vi "Save Animated GIF To File (Core).vi"(7 "Dither (None)":T2, 8 "error in (no error)":errorcluster, 9 "Delays":i32[](array[numeric]), 10 "Frames":T1[](array[typedef]), 11 "Path In":string) -> (0 "error out":errorcluster, 3 "Path Out":string)   [LabVIEW 2020, in "G-Image.lvlib"]
doc: "Saves an image in GIF format to disk."
uses:
  G-Image.lvlib
  Controls/Dither Type.ctl
  <vilib>/picture/picture.llb/imagedata.ctl
  Private/ARGB To RGBA.vi
  Private/Depth To Number Channels.vi
  <vilib>/Utility/error.llb/Error Cluster From Error Code.vi
  lib/g_image_32.dll
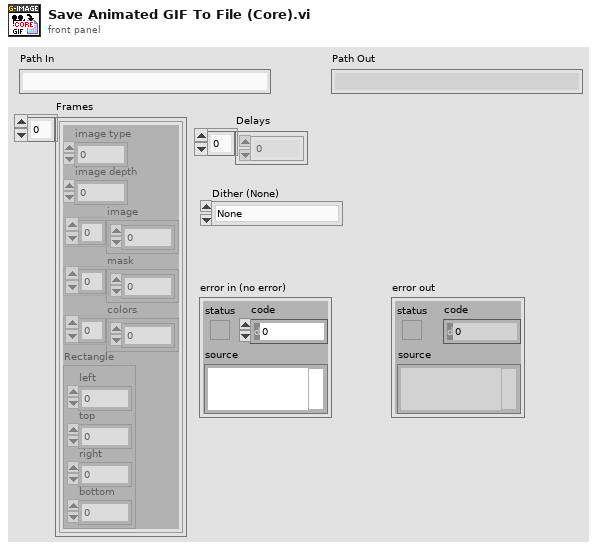
[diagram p1: front panel]
types:
  T1 = typedef "imagedata.ctl" = cluster{"image type":i32, "image depth":i32, "image":u8[], "mask":u8[], "colors":u32[], "Rectangle":cluster{"left":i16, "top":i16, "right":i16, "bottom":i16}}
  T2 = typedef "G-Image.lvlib/Dither Type.ctl" = enum32{"None", "Floyd-Steinberg"}
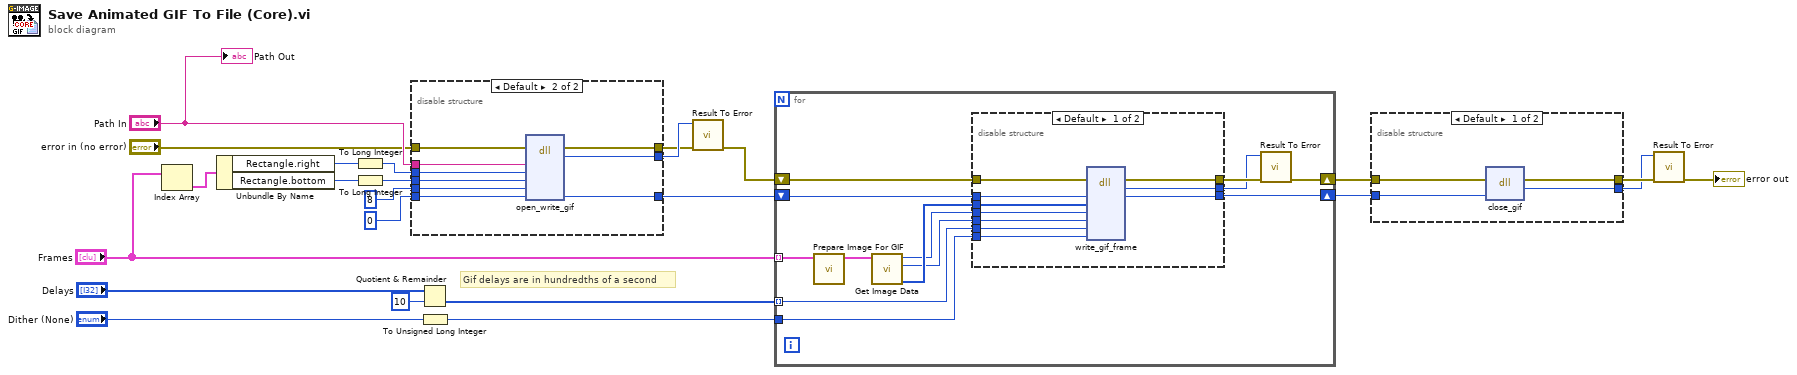
[diagram p0: block diagram]
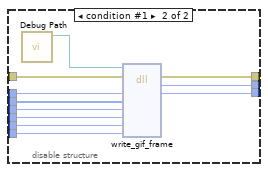
[diagram p2: hidden frame]
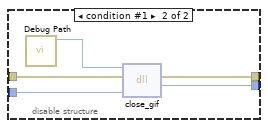
[diagram p3: hidden frame]
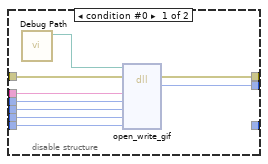
[diagram p4: hidden frame]
diagram:
  # "Gif delays are in hundredths of a second"
  n1 = Index Array(array="Frames") -> (element=w21:T1)  [unwired: 1 in]
  n2 = Unbundle By Name(w21) -> ("Rectangle.right"=w20:i16, "Rectangle.bottom"=w18:i16)
  n3 = To Long Integer(number=w20) -> (32bit integer=w19:i32)
  n4 = To Long Integer(number=w18) -> (32bit integer=w17:i32)
  n5 = disable-structure shown="Default" {
    disable-tunnel: [w33 w42] -> w22
    disable-tunnel: "error in (no error)" -> [w32 w41]
    disable-tunnel: [w31 w40] -> w23
    disable-tunnel: "Path In" -> [w29 w39]
    disable-tunnel: w19 -> [w28 w38]
    disable-tunnel: w17 -> [w27 w37]
    disable-tunnel: 8 -> [w26 w36]
    disable-tunnel: i64 0 ("writer_ptr") -> [w25 w35]
    disable-tunnel: [_ w34] -> w12
    frame condition #0 {
      n6 = call "Debug Path.vi"() -> ("Debug Path"=w30:path)  [unwired: 11 in]
      n7 = dll-call lib="?" fn="open_write_gif"(path in=w30, error in=w32, "file_name"=w29, "width"=w28, "height"=w27, "depth"=w26, "writer_ptr"=w25) -> (error out=w33:errorcluster, "result"=w31:i32)  [unwired: 6 in, 1 out]
    }
    frame condition #1 (active) {
      n8 = dll-call lib="C:/github/dataflowg/g-image/src/LabVIEW/G-Image/lib/g_image_*.*" fn="open_write_gif"(error in=w41, "file_name"=w39, "width"=w38, "height"=w37, "depth"=w36, "writer_ptr"=w35) -> (error out=w42:errorcluster, "result"=w40:i32, "writer_ptr"=w34:i64)  [unwired: 6 in, 1 out]
    }
  }
  n9 = Quotient & Remainder(x="Delays", y=10) -> (floor(x/y)=w1:i32[])  [unwired: 1 out]
  n10 = To Unsigned Long Integer(number="Dither (None)") -> (unsigned 32bit integer=w9:u32)
  n11 = call "Result To Error.vi"("error in (no error)"=w22, "Result Code"=w23) -> ("error out"=w8:errorcluster)  [unwired: 9 in]
  n12 = for {
    shift-right: [w54] -> w6
    shift-left: w12 -> [w55]
    tunnel: "Frames" -> [w47] mode=indexing
    tunnel: w1 -> [w53] mode=indexing
    tunnel: w9 -> [w52]
    shift-right: [w49] -> w7
    shift-left: w8 -> [w48]
    n13 = call "Prepare Image For GIF.vi"("Image"=w47) -> ("Image"=w46:T1)  [unwired: 9 in, 1 out]
    n14 = call "Get Image Data.vi"("Image"=w46) -> ("Image (RGBA)"=w45:u8[], "Height"=w43:i32, "Width"=w44:i32)  [unwired: 7 in, 1 out]
    n15 = disable-structure shown="Default" {
      disable-tunnel: [w65 w76] -> w51
      disable-tunnel: w48 -> [w64 w75]
      disable-tunnel: [w63 w74] -> w50
      disable-tunnel: w55 -> [w62 w73]
      disable-tunnel: w45 -> [w60 w71]
      disable-tunnel: w44 -> [w59 w70]
      disable-tunnel: w43 -> [w58 w69]
      disable-tunnel: w53 -> [w57 w68]
      disable-tunnel: [w61 w72] -> w54
      disable-tunnel: w52 -> [w56 w67]
      frame condition #0 (active) {
        n16 = dll-call lib="C:/github/dataflowg/g-image/src/LabVIEW/G-Image/lib/g_image_*.*" fn="write_gif_frame"(error in=w64, "writer_ptr"=w62, "image_data"=w60, "width"=w59, "height"=w58, "delay"=w57, "dither"=w56) -> (error out=w65:errorcluster, "result"=w63:i32, "writer_ptr"=w61:i64)  [unwired: 7 in, 1 out]
      }
      frame condition #1 {
        n17 = call "Debug Path.vi"() -> ("Debug Path"=w66:path)  [unwired: 11 in]
        n18 = dll-call lib="?" fn="write_gif_frame"(path in=w66, error in=w75, "writer_ptr"=w73, "image_data"=w71, "width"=w70, "height"=w69, "delay"=w68, "dither"=w67) -> (error out=w76:errorcluster, "result"=w74:i32, "writer_ptr"=w72:i64)  [unwired: 6 in, 1 out]
      }
    }
    n19 = call "Result To Error.vi"("error in (no error)"=w51, "Result Code"=w50) -> ("error out"=w49:errorcluster)  [unwired: 9 in]
  }
  n20 = disable-structure shown="Default" {
    disable-tunnel: [w80 w85] -> w5
    disable-tunnel: w7 -> [w79 w84]
    disable-tunnel: [w78 w83] -> w3
    disable-tunnel: w6 -> [w77 w82]
    frame condition #0 (active) {
      n21 = dll-call lib="C:/github/dataflowg/g-image/src/LabVIEW/G-Image/lib/g_image_*.*" fn="close_gif"(error in=w79, "writer_ptr"=w77) -> (error out=w80:errorcluster, "result"=w78:i32)  [unwired: 3 in, 1 out]
    }
    frame condition #1 {
      n22 = call "Debug Path.vi"() -> ("Debug Path"=w81:path)  [unwired: 11 in]
      n23 = dll-call lib="?" fn="close_gif"(path in=w81, error in=w84, "writer_ptr"=w82) -> (error out=w85:errorcluster, "result"=w83:i32)  [unwired: 2 in, 1 out]
    }
  }
  n24 = call "Result To Error.vi"("error in (no error)"=w5, "Result Code"=w3) -> ("error out"=→"error out":errorcluster)  [unwired: 9 in]
  "Path Out" <- "Path In"
